vi "ttm_tensilecyclic_poller.vi"() -> ()   [LabVIEW 2011]
panel:
  out "error out":errorcluster
  out "Cycles":i32
  out "Afterramp":i32
  out "Preramp":i32
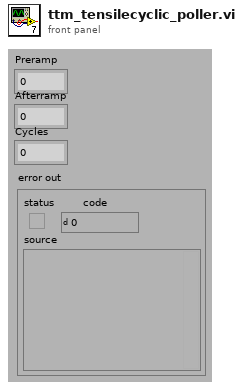
[diagram p1: front panel]
types:
  T1 = cluster{"Name":string, "Type":i32, "SI Full Scale":dbl, "Full Scale":dbl, "Units String":string, "Display Format":string, "Gauge Length":dbl}[][]
  T2 = cluster{"Device ID":i32, "Device Name":string, "Device Type":i32}[]
  T3 = cluster{"Double":dbl, "Set Point Time":dbl, "Double":dbl, "Double":dbl}
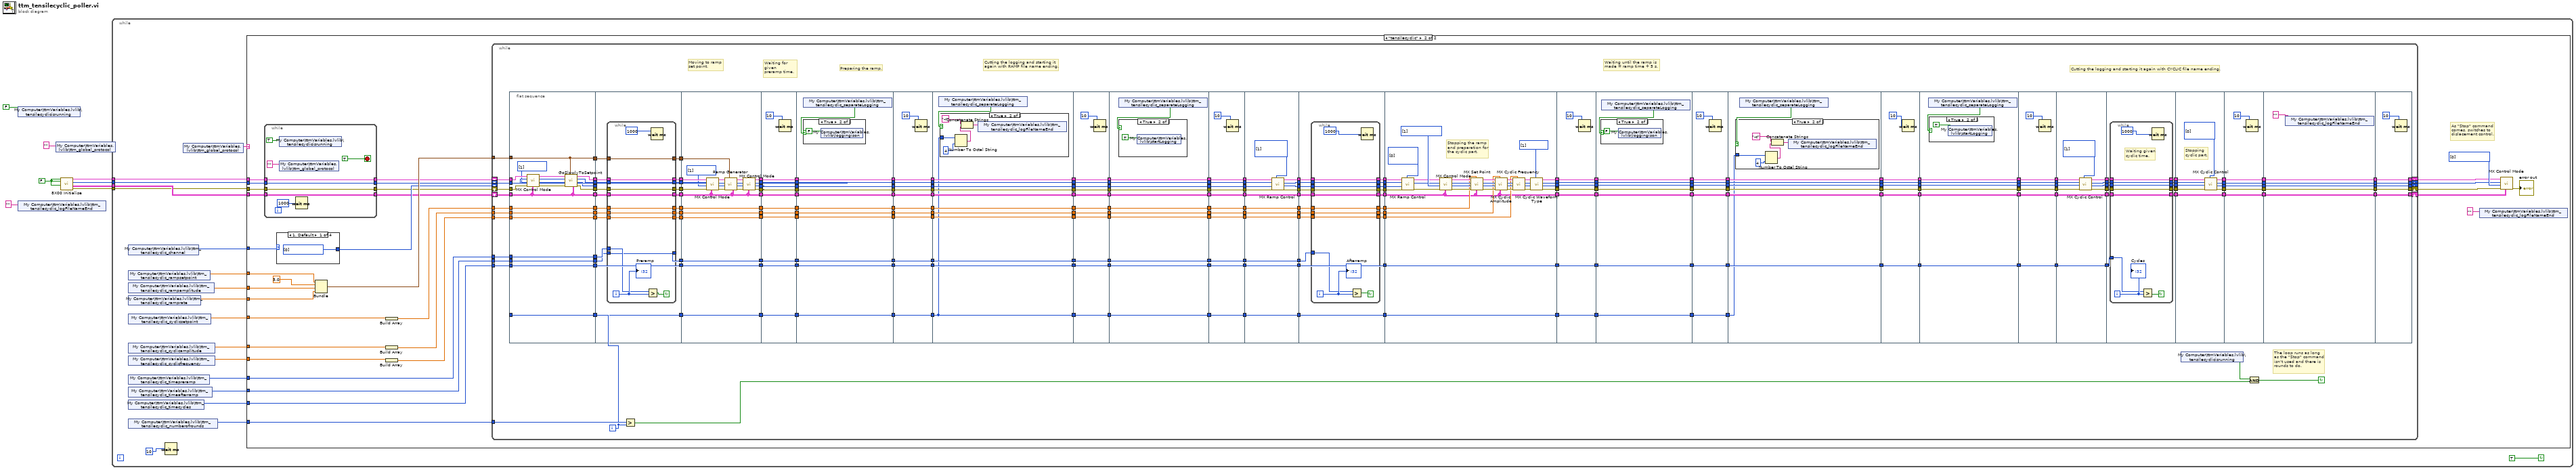
[diagram p0: block diagram]
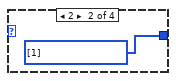
[diagram p9: hidden frame]
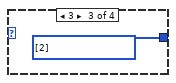
[diagram p10: hidden frame]
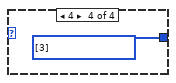
[diagram p11: hidden frame]
diagram:
  w4 = FALSE ("Reset?")
  n1 = shared-variable "My Computer\\ttmVariables.lvlib\\tensilecyclicisrunning"(FALSE ("tensilecyclicisrunning")) -> ()  [unwired: 1 in, 1 out]
  n2 = shared-variable "My Computer\\ttmVariables.lvlib\\ttm_tensilecyclic_logFileNameEnd"("" ("protocol")) -> ()  [unwired: 1 in, 1 out]
  n3 = shared-variable "My Computer\\ttmVariables.lvlib\\ttm_global_protocol"("" ("protocol")) -> ()  [unwired: 1 in, 1 out]
  n4 = call "8X00 Initialise.vi"("Reset?"=w4, "Create DVM? (T)"=w4, "Create Console? (T)"=w4) -> ("error out"=w5:errorcluster, "Channel Data"=w8:T1, "Axis Selector"=w6:i32[], "Axis Information"=w7:T2)  [unwired: 1 in]
  n5 = while {
    tunnel: w8 -> [w24]
    tunnel: w7 -> [w25]
    tunnel: w6 -> [w13]
    tunnel: w5 -> [w23]
    stop <- TRUE continue-if-true
    n6 = shared-variable "My Computer\\ttmVariables.lvlib\\ttm_tensilecyclic_channel"() -> (w19:i32)  [unwired: 1 in, 1 out]
    n7 = shared-variable "My Computer\\ttmVariables.lvlib\\ttm_tensilecyclic_rampsetpoint"() -> (w12:dbl)  [unwired: 1 in, 1 out]
    n8 = shared-variable "My Computer\\ttmVariables.lvlib\\ttm_tensilecyclic_rampamplitude"() -> (w22:dbl)  [unwired: 1 in, 1 out]
    n9 = shared-variable "My Computer\\ttmVariables.lvlib\\ttm_tensilecyclic_ramprate"() -> (w21:dbl)  [unwired: 1 in, 1 out]
    n10 = shared-variable "My Computer\\ttmVariables.lvlib\\ttm_tensilecyclic_cyclicsetpoint"() -> (w17:dbl)  [unwired: 1 in, 1 out]
    n11 = shared-variable "My Computer\\ttmVariables.lvlib\\ttm_tensilecyclic_cyclicamplitude"() -> (w16:dbl)  [unwired: 1 in, 1 out]
    n12 = shared-variable "My Computer\\ttmVariables.lvlib\\ttm_tensilecyclic_cyclicfrequency"() -> (w15:dbl)  [unwired: 1 in, 1 out]
    n13 = shared-variable "My Computer\\ttmVariables.lvlib\\ttm_tensilecyclic_timepreramp"() -> (w11:i32)  [unwired: 1 in, 1 out]
    n14 = shared-variable "My Computer\\ttmVariables.lvlib\\ttm_tensilecyclic_timeafterramp"() -> (w9:i32)  [unwired: 1 in, 1 out]
    n15 = shared-variable "My Computer\\ttmVariables.lvlib\\ttm_tensilecyclic_timecycles"() -> (w10:i32)  [unwired: 1 in, 1 out]
    n16 = shared-variable "My Computer\\ttmVariables.lvlib\\ttm_tensilecyclic_numberofrounds"() -> (w14:i32)  [unwired: 1 in, 1 out]
    n17 = Wait (ms)(milliseconds to wait=u32 10) -> ()  [unwired: 1 out]
    n18 = shared-variable "My Computer\\ttmVariables.lvlib\\ttm_global_protocol"() -> (w18:string)  [unwired: 1 in, 1 out]
    n19 = case shown="\"tensilecyclic\"" w18 {
      tunnel: w13 -> [_ w46]
      tunnel: w25 -> [_ w47]
      tunnel: w24 -> [_ w44]
      tunnel: w23 -> [_ w45]
      tunnel: w22 -> [_ w57]
      tunnel: w21 -> [_ w56]
      tunnel: w19 -> [_ w55]
      tunnel: w17 -> [_ w54]
      tunnel: w16 -> [_ w52]
      tunnel: w15 -> [_ w49]
      tunnel: w14 -> [_ w43]
      tunnel: w12 -> [_ w32]
      tunnel: w11 -> [_ w31]
      tunnel: w10 -> [_ w30]
      tunnel: w9 -> [_ w29]
      frame "", Default {
      }
      frame "tensilecyclic" {
        w37 = u16[] [0] items=["Channel 1", "Channel 2", "Channel 3", "Channel 4"] ("Control Modes")
        # "As \"Stop\" command\ncomes, switches to\ndislacement control."
        n20 = while {
          tunnel: [w62] -> w42
          tunnel: w47 -> [w62]
          tunnel: [w61] -> w41
          tunnel: w46 -> [w61]
          tunnel: [w60] -> w39
          tunnel: w45 -> [w60]
          tunnel: [w59] -> w38
          tunnel: w44 -> [w59]
          stop <- TRUE stop-if-true
          n21 = shared-variable "My Computer\\ttmVariables.lvlib\\tensilecyclicisrunning"(TRUE ("tensilecyclicisrunning")) -> ()  [unwired: 1 in, 1 out]
          n22 = shared-variable "My Computer\\ttmVariables.lvlib\\ttm_global_protocol"("" ("protocol")) -> ()  [unwired: 1 in, 1 out]
          n23 = Wait (ms)(milliseconds to wait=u32 1000) -> ()  [unwired: 1 out]
        }
        n24 = case shown="1, Default" w55 {
          tunnel: [w671 w672 w673 w674] -> w40
          frame 1, Default {
            w671 = u16[] [0] items=["Channel 1", "Channel 2", "Channel 3", "Channel 4"] ("Choose channel to apply\nthe setpoint")
          }
          frame 2 {
            w672 = u16[] [1] items=["Channel 1", "Channel 2", "Channel 3", "Channel 4"] ("Choose channel to apply\nthe setpoint")
          }
          frame 3 {
            w673 = u16[] [2] items=["Channel 1", "Channel 2", "Channel 3", "Channel 4"] ("Choose channel to apply\nthe setpoint")
          }
          frame 4 {
            w674 = u16[] [3] items=["Channel 1", "Channel 2", "Channel 3", "Channel 4"] ("Choose channel to apply\nthe setpoint")
          }
        }
        n25 = Bundle("Double"=w32, "Set Point Time"=3.0, "Double"=w57, "Double"=w56) -> (w58:T3)  [unwired: 1 in]
        n26 = Build Array(w54) -> (w53:dbl[])
        n27 = Build Array(w52) -> (w51:dbl[])
        n28 = Build Array(w49) -> (w48:dbl[])
        n29 = while {
          tunnel: w58 -> [w84]
          tunnel: w53 -> [w79]
          tunnel: w51 -> [w78]
          tunnel: w48 -> [w77]
          tunnel: w43 -> [w298]
          shift-right: [w72] -> w36
          shift-left: w42 -> [w83]
          shift-right: [w71] -> w35
          shift-left: w41 -> [w82]
          shift-right: [w70] -> _
          shift-left: w40 -> [_]
          shift-right: [w69] -> w34
          shift-left: w39 -> [w81]
          shift-right: [w68] -> w33
          shift-left: w38 -> [w80]
          tunnel: w31 -> [w76]
          tunnel: w29 -> [w74]
          tunnel: w30 -> [w73]
          i -> [w75]
          stop <- w67 continue-if-true
          # "Waiting until the ramp is made = ramp time + 5 s."
          # "Moving to ramp\nset point."
          # "Waiting for given\npreramp time."
          # "Preparing the ramp."
          # "Cutting the logging and starting it again with RAMP file name ending."
          # "Cutting the logging and starting it again with CYCLIC file name ending."
          # "The loop runs as long\nas the \"Stop\" command\nisn't used and there is \nrounds to do."
          n30 = flat-sequence {
            tunnel: w84 -> [w303]
            tunnel: w82 -> [w316]
            tunnel: w83 -> [w317]
            tunnel: w79 -> [w319]
            tunnel: w78 -> [w318]
            tunnel: [w319] -> w295
            tunnel: [w318] -> w294
            tunnel: [w310] -> w293
            tunnel: [w309] -> w292
            tunnel: [w308] -> w291
            tunnel: [w307] -> w290
            tunnel: [w304] -> w289
            tunnel: [w303] -> w288
            tunnel: w77 -> [w306]
            tunnel: [w306] -> w287
            tunnel: w81 -> [w305]
            tunnel: w80 -> [w304]
            tunnel: w76 -> [w302]
            tunnel: [w302] -> w286
            tunnel: w74 -> [w301]
            tunnel: [w301] -> w285
            tunnel: w73 -> [w300]
            tunnel: [w300] -> w284
            tunnel: [w299] -> w283
            tunnel: w75 -> [w299]
            tunnel: w295 -> [w330]
            tunnel: [w329] -> w282
            tunnel: w294 -> [w327]
            tunnel: [w328] -> w281
            tunnel: w293 -> [w337]
            tunnel: [w338] -> w280
            tunnel: w292 -> [w336]
            tunnel: [w335] -> w279
            tunnel: w291 -> [_]
            tunnel: w290 -> [w333]
            tunnel: [w334] -> w278
            tunnel: w289 -> [w331]
            tunnel: [w332] -> w277
            tunnel: [w339] -> w276
            tunnel: w288 -> [w340]
            tunnel: [w326] -> w275
            tunnel: w287 -> [w325]
            tunnel: w286 -> [w324]
            tunnel: [w323] -> w274
            tunnel: w285 -> [w322]
            tunnel: w284 -> [w321]
            tunnel: [w321] -> w273
            tunnel: [w320] -> w272
            tunnel: w283 -> [w320]
            tunnel: w282 -> [w377]
            tunnel: [w377] -> w271
            tunnel: w281 -> [w376]
            tunnel: [w376] -> w270
            tunnel: w280 -> [w367]
            tunnel: [w358] -> w269
            tunnel: w279 -> [w366]
            tunnel: [w357] -> w268
            tunnel: [w355] -> w267
            tunnel: w278 -> [w364]
            tunnel: [w356] -> w266
            tunnel: w277 -> [w362]
            tunnel: [w362] -> w265
            tunnel: w276 -> [w363]
            tunnel: w275 -> [w361]
            tunnel: [w361] -> w264
            tunnel: [w360] -> w263
            tunnel: w274 -> [w360]
            tunnel: [w359] -> w262
            tunnel: w273 -> [w359]
            tunnel: [w354] -> w261
            tunnel: w272 -> [w354]
            tunnel: w271 -> [w389]
            tunnel: [w389] -> w260
            tunnel: w270 -> [w388]
            tunnel: [w388] -> w259
            tunnel: w269 -> [w387]
            tunnel: [w387] -> w258
            tunnel: w268 -> [w386]
            tunnel: [w386] -> w257
            tunnel: w267 -> [w385]
            tunnel: [w385] -> w256
            tunnel: w266 -> [w384]
            tunnel: [w384] -> w255
            tunnel: w265 -> [w383]
            tunnel: [w383] -> w254
            tunnel: w264 -> [w382]
            tunnel: [w382] -> w253
            tunnel: w263 -> [w381]
            tunnel: [w381] -> w252
            tunnel: w262 -> [w380]
            tunnel: [w380] -> w251
            tunnel: w261 -> [w379]
            tunnel: [w379] -> w250
            tunnel: w260 -> [w401]
            tunnel: [w401] -> w249
            tunnel: w259 -> [w400]
            tunnel: [w400] -> w248
            tunnel: w258 -> [w399]
            tunnel: [w399] -> w247
            tunnel: w257 -> [w398]
            tunnel: [w398] -> w246
            tunnel: w256 -> [w397]
            tunnel: [w397] -> w245
            tunnel: w255 -> [w396]
            tunnel: [w396] -> w244
            tunnel: w254 -> [w395]
            tunnel: [w395] -> w243
            tunnel: w253 -> [w394]
            tunnel: [w394] -> w242
            tunnel: w252 -> [w393]
            tunnel: [w393] -> w241
            tunnel: w251 -> [w392]
            tunnel: [w392] -> w240
            tunnel: [w391] -> w239
            tunnel: w250 -> [w391]
            tunnel: w249 -> [w414]
            tunnel: [w414] -> w238
            tunnel: w248 -> [w413]
            tunnel: [w413] -> w237
            tunnel: w247 -> [w412]
            tunnel: [w412] -> w236
            tunnel: w246 -> [w411]
            tunnel: [w411] -> w235
            tunnel: w245 -> [w410]
            tunnel: [w410] -> w234
            tunnel: w244 -> [w409]
            tunnel: [w409] -> w233
            tunnel: w243 -> [w408]
            tunnel: [w408] -> w232
            tunnel: w242 -> [w407]
            tunnel: [w407] -> w231
            tunnel: w241 -> [w406]
            tunnel: [w406] -> w230
            tunnel: w240 -> [w405]
            tunnel: [w405] -> w229
            tunnel: [w404] -> w228
            tunnel: w239 -> [w404]
            tunnel: w238 -> [w426]
            tunnel: [w426] -> w227
            tunnel: w237 -> [w425]
            tunnel: [w425] -> w226
            tunnel: w236 -> [w424]
            tunnel: [w424] -> w225
            tunnel: w235 -> [w423]
            tunnel: [w423] -> w224
            tunnel: w234 -> [w422]
            tunnel: [w422] -> w223
            tunnel: w233 -> [w421]
            tunnel: [w421] -> w222
            tunnel: w232 -> [w420]
            tunnel: [w420] -> w221
            tunnel: w231 -> [w419]
            tunnel: [w419] -> w220
            tunnel: w230 -> [w418]
            tunnel: [w418] -> w219
            tunnel: w229 -> [w417]
            tunnel: [w417] -> w218
            tunnel: w228 -> [w415]
            tunnel: [w415] -> w217
            tunnel: w227 -> [w443]
            tunnel: [w443] -> w216
            tunnel: w226 -> [w442]
            tunnel: [w442] -> w215
            tunnel: w225 -> [w441]
            tunnel: [w441] -> w214
            tunnel: w224 -> [w440]
            tunnel: [w440] -> w213
            tunnel: w223 -> [w439]
            tunnel: [w439] -> w212
            tunnel: w222 -> [w438]
            tunnel: [w438] -> w211
            tunnel: w221 -> [w437]
            tunnel: [w437] -> w210
            tunnel: w220 -> [w436]
            tunnel: [w436] -> w209
            tunnel: w219 -> [w435]
            tunnel: [w435] -> w208
            tunnel: w218 -> [w434]
            tunnel: [w434] -> w207
            tunnel: [w433] -> w206
            tunnel: w217 -> [w433]
            tunnel: w216 -> [w455]
            tunnel: [w455] -> w205
            tunnel: w215 -> [w454]
            tunnel: [w454] -> w204
            tunnel: w214 -> [w453]
            tunnel: [w453] -> w203
            tunnel: w213 -> [w452]
            tunnel: [w452] -> w202
            tunnel: w212 -> [w451]
            tunnel: [w451] -> w201
            tunnel: w211 -> [w450]
            tunnel: [w450] -> w200
            tunnel: w210 -> [w449]
            tunnel: [w449] -> w199
            tunnel: w209 -> [w448]
            tunnel: [w448] -> w198
            tunnel: w208 -> [w447]
            tunnel: [w447] -> w197
            tunnel: w207 -> [w446]
            tunnel: [w446] -> w196
            tunnel: [w445] -> w195
            tunnel: w206 -> [w445]
            tunnel: w205 -> [w468]
            tunnel: [w468] -> w194
            tunnel: w204 -> [w467]
            tunnel: [w467] -> w193
            tunnel: w203 -> [w466]
            tunnel: [w466] -> w192
            tunnel: w202 -> [w465]
            tunnel: [w465] -> w191
            tunnel: w201 -> [w464]
            tunnel: [w464] -> w190
            tunnel: w200 -> [w463]
            tunnel: [w463] -> w189
            tunnel: w199 -> [w462]
            tunnel: [w462] -> w188
            tunnel: w198 -> [w461]
            tunnel: [w461] -> w187
            tunnel: w197 -> [w460]
            tunnel: [w460] -> w186
            tunnel: w196 -> [w459]
            tunnel: [w459] -> w185
            tunnel: [w458] -> w184
            tunnel: w195 -> [w458]
            tunnel: w194 -> [w484]
            tunnel: [w484] -> w183
            tunnel: w193 -> [w483]
            tunnel: [w483] -> w182
            tunnel: w192 -> [w471]
            tunnel: [w478] -> w181
            tunnel: w191 -> [w472]
            tunnel: [w477] -> w180
            tunnel: w190 -> [w473]
            tunnel: [w476] -> w179
            tunnel: w189 -> [w474]
            tunnel: [w475] -> w178
            tunnel: w188 -> [w470]
            tunnel: [w470] -> w177
            tunnel: w187 -> [w482]
            tunnel: [w482] -> w176
            tunnel: w186 -> [w481]
            tunnel: [w481] -> w175
            tunnel: w185 -> [w480]
            tunnel: [w480] -> w174
            tunnel: [w469] -> w173
            tunnel: w184 -> [w469]
            tunnel: [w493] -> w172
            tunnel: w183 -> [w492]
            tunnel: [w491] -> w171
            tunnel: w182 -> [w490]
            tunnel: [w503] -> w170
            tunnel: w181 -> [w502]
            tunnel: [w501] -> w169
            tunnel: w180 -> [w500]
            tunnel: [w499] -> w168
            tunnel: w179 -> [w498]
            tunnel: [w497] -> w167
            tunnel: w178 -> [w496]
            tunnel: [w495] -> w166
            tunnel: w177 -> [w494]
            tunnel: [w488] -> w165
            tunnel: w176 -> [w489]
            tunnel: w175 -> [w487]
            tunnel: w174 -> [w486]
            tunnel: [w486] -> w164
            tunnel: [w485] -> w163
            tunnel: w173 -> [w485]
            tunnel: w172 -> [w546]
            tunnel: w171 -> [w529]
            tunnel: w170 -> [w545]
            tunnel: w169 -> [w544]
            tunnel: w168 -> [w543]
            tunnel: w167 -> [w542]
            tunnel: w166 -> [w523]
            tunnel: [w519] -> w162
            tunnel: [w518] -> w161
            tunnel: [w517] -> w160
            tunnel: [w516] -> w159
            tunnel: w165 -> [w524]
            tunnel: [w523] -> w158
            tunnel: w164 -> [w522]
            tunnel: [w522] -> w157
            tunnel: [w520] -> w156
            tunnel: w163 -> [w520]
            tunnel: w162 -> [w559]
            tunnel: [w559] -> w155
            tunnel: w161 -> [w558]
            tunnel: [w558] -> w154
            tunnel: w160 -> [w557]
            tunnel: [w557] -> w153
            tunnel: w159 -> [w556]
            tunnel: [w556] -> w152
            tunnel: w158 -> [w555]
            tunnel: [w555] -> w151
            tunnel: w157 -> [w554]
            tunnel: [w554] -> w150
            tunnel: w156 -> [w553]
            tunnel: [w553] -> w149
            tunnel: w155 -> [w567]
            tunnel: [w567] -> w148
            tunnel: w154 -> [w566]
            tunnel: [w566] -> w147
            tunnel: w153 -> [w565]
            tunnel: [w565] -> w146
            tunnel: w152 -> [w564]
            tunnel: [w564] -> w145
            tunnel: w151 -> [w563]
            tunnel: [w563] -> w144
            tunnel: w150 -> [w562]
            tunnel: [w562] -> w143
            tunnel: w149 -> [w561]
            tunnel: [w561] -> w142
            tunnel: w148 -> [w576]
            tunnel: [w576] -> w141
            tunnel: w147 -> [w575]
            tunnel: [w575] -> w140
            tunnel: w146 -> [w574]
            tunnel: [w574] -> w139
            tunnel: w145 -> [w573]
            tunnel: [w573] -> w138
            tunnel: w144 -> [w572]
            tunnel: [w572] -> w137
            tunnel: w143 -> [w571]
            tunnel: [w571] -> w136
            tunnel: w142 -> [w570]
            tunnel: [w570] -> w135
            tunnel: w141 -> [w584]
            tunnel: [w584] -> w134
            tunnel: w140 -> [w583]
            tunnel: [w583] -> w133
            tunnel: w139 -> [w582]
            tunnel: [w582] -> w132
            tunnel: w138 -> [w581]
            tunnel: [w581] -> w131
            tunnel: w137 -> [w580]
            tunnel: [w580] -> w130
            tunnel: w136 -> [w579]
            tunnel: [w579] -> w129
            tunnel: w135 -> [w577]
            tunnel: w134 -> [w596]
            tunnel: [w596] -> w128
            tunnel: w133 -> [w595]
            tunnel: [w595] -> w127
            tunnel: w132 -> [w594]
            tunnel: [w594] -> w126
            tunnel: w131 -> [w593]
            tunnel: [w593] -> w125
            tunnel: w130 -> [w592]
            tunnel: [w592] -> w124
            tunnel: w129 -> [w591]
            tunnel: [w591] -> w123
            tunnel: w128 -> [w603]
            tunnel: [w603] -> w122
            tunnel: w127 -> [w602]
            tunnel: [w602] -> w121
            tunnel: w126 -> [w601]
            tunnel: [w601] -> w120
            tunnel: w125 -> [w600]
            tunnel: [w600] -> w119
            tunnel: w124 -> [w599]
            tunnel: [w599] -> w118
            tunnel: w123 -> [w598]
            tunnel: [w598] -> w117
            tunnel: w122 -> [w611]
            tunnel: [w611] -> w116
            tunnel: w121 -> [w610]
            tunnel: [w610] -> w115
            tunnel: w120 -> [w609]
            tunnel: [w609] -> w114
            tunnel: w119 -> [w608]
            tunnel: [w608] -> w113
            tunnel: w118 -> [w607]
            tunnel: [w607] -> w112
            tunnel: w117 -> [w606]
            tunnel: [w606] -> w111
            tunnel: w116 -> [w617]
            tunnel: [w619] -> w110
            tunnel: w115 -> [w616]
            tunnel: [w618] -> w109
            tunnel: w114 -> [w615]
            tunnel: w113 -> [w614]
            tunnel: [w612] -> w108
            tunnel: w112 -> [w622]
            tunnel: [w622] -> w107
            tunnel: w111 -> [w621]
            tunnel: [w621] -> w106
            tunnel: [w613] -> w105
            tunnel: w110 -> [w632]
            tunnel: [w633] -> w104
            tunnel: [w631] -> w103
            tunnel: w109 -> [w630]
            tunnel: [w629] -> w102
            tunnel: [w627] -> w101
            tunnel: w108 -> [w626]
            tunnel: [w625] -> w100
            tunnel: w107 -> [w624]
            tunnel: w106 -> [w623]
            tunnel: w105 -> [w628]
            tunnel: w104 -> [w652]
            tunnel: w103 -> [w651]
            tunnel: w102 -> [w650]
            tunnel: w101 -> [w649]
            tunnel: w100 -> [w643]
            tunnel: [w647] -> w99
            tunnel: [w646] -> w98
            tunnel: [w645] -> w97
            tunnel: [w644] -> w96
            tunnel: [w643] -> w95
            tunnel: w99 -> [w658]
            tunnel: w98 -> [w657]
            tunnel: w97 -> [w656]
            tunnel: w96 -> [w655]
            tunnel: w95 -> [w654]
            tunnel: [w658] -> w94
            tunnel: [w657] -> w93
            tunnel: [w656] -> w92
            tunnel: [w655] -> w91
            tunnel: [w654] -> w90
            tunnel: w94 -> [w664]
            tunnel: w93 -> [w663]
            tunnel: w92 -> [w662]
            tunnel: w91 -> [w661]
            tunnel: w90 -> [w660]
            tunnel: [w664] -> w89
            tunnel: [w663] -> w88
            tunnel: [w662] -> w87
            tunnel: [w661] -> w86
            tunnel: [w660] -> w85
            tunnel: [w666] -> w68
            tunnel: [w667] -> w69
            tunnel: [w668] -> w70
            tunnel: [w669] -> w71
            tunnel: [w670] -> w72
            tunnel: w89 -> [w670]
            tunnel: w88 -> [w669]
            tunnel: w87 -> [w668]
            tunnel: w86 -> [w667]
            tunnel: w85 -> [w666]
            frame #0 {
              w311 = u16[] [1] items=["Channel 1", "Channel 2", "Channel 3", "Channel 4"] ("Control Modes")
              n31 = call "MX Control Mode.vi"("Channel Data"=w304, "error in (no error)"=w305, "Control Modes"=w311, "Axis Selector"=w316, "Axis Information"=w317) -> ("error out"=w315:errorcluster, "Control Modes out"=w314:u16[], "Axis Selector out"=w313:i32[], "Axis Information out"=w312:T2)  [unwired: 1 in]
              n32 = call "GoSlowlyToSetpoint.vi"("Channel Data"=w304, "Input cluster"=w303, "error in (no error)"=w315, "Channels"=w314, "Axis Selector"=w313, "Axis Information"=w312) -> ("Error Out"=w307:errorcluster, "Channels Out"=w308:u16[], "Axis Selector Out"=w309:i32[], "Axis Information Out"=w310:T2)  [unwired: 2 in]
            }
            frame #1 {
              n33 = while {
                tunnel: w340 -> [w352]
                tunnel: [w352] -> w339
                tunnel: [w351] -> w338
                tunnel: w337 -> [w351]
                tunnel: w336 -> [w350]
                tunnel: [w350] -> w335
                tunnel: [w349] -> w334
                tunnel: w333 -> [w349]
                tunnel: [w348] -> w332
                tunnel: w331 -> [w348]
                tunnel: [w347] -> w329
                tunnel: w330 -> [w347]
                tunnel: [w346] -> w328
                tunnel: w327 -> [w346]
                tunnel: [w345] -> w326
                tunnel: w325 -> [w345]
                tunnel: w324 -> [w342]
                tunnel: [w341] -> w323
                tunnel: w322 -> [w341]
                i -> [w343]
                stop <- w344 continue-if-true
                n34 = Greater?(x=w342, y=w343) -> (0:w344:bool)
                n35 = Wait (ms)(milliseconds to wait=u32 1000) -> ()  [unwired: 1 out]
                "Preramp" <- w343
              }
            }
            frame #2 {
              w365 = u16[] [1] items=["Channel 1", "Channel 2", "Channel 3", "Channel 4"] ("Control Modes")
              n36 = call "MX Control Mode.vi"("Channel Data"=w362, "error in (no error)"=w364, "Control Modes"=w365, "Axis Selector"=w366, "Axis Information"=w367) -> ("error out"=w368:errorcluster, "Control Modes out"=w369:u16[], "Axis Selector out"=w370:i32[], "Axis Information out"=w371:T2)  [unwired: 1 in]
              n37 = call "Ramp Generator.vi"("Channel Data"=w362, "Input cluster"=w363, "error in (no error)"=w368, "Channels"=w369, "Axis Selector"=w370, "Axis Information"=w371) -> ("Error Out"=w372:errorcluster, "Channels Out"=w373:u16[], "Axis Selector Out"=w374:i32[], "Axis Information Out"=w375:T2)  [unwired: 2 in]
              n38 = call "MX Control Mode.vi"("Channel Data"=w362, "error in (no error)"=w372, "Control Modes"=w373, "Axis Selector"=w374, "Axis Information"=w375) -> ("error out"=w356:errorcluster, "Control Modes out"=w355:u16[], "Axis Selector out"=w357:i32[], "Axis Information out"=w358:T2)  [unwired: 1 in]
            }
            frame #3 {
              n39 = Wait (ms)(milliseconds to wait=u32 10) -> ()  [unwired: 1 out]
            }
            frame #4 {
              n40 = shared-variable "My Computer\\ttmVariables.lvlib\\ttm_tensilecyclic_separateLogging"() -> (w390:bool)  [unwired: 1 in, 1 out]
              n41 = case shown="True" w390 {
                frame False {
                }
                frame True {
                  n42 = shared-variable "My Computer\\ttmVariables.lvlib\\loggingison"(FALSE ("tensilecyclicisrunning")) -> ()  [unwired: 1 in, 1 out]
                }
              }
            }
            frame #5 {
              n43 = Wait (ms)(milliseconds to wait=u32 10) -> ()  [unwired: 1 out]
            }
            frame #6 {
              n44 = shared-variable "My Computer\\ttmVariables.lvlib\\ttm_tensilecyclic_separateLogging"() -> (w416:bool)  [unwired: 1 in, 1 out]
              n45 = case shown="True" w416 {
                tunnel: w415 -> [_ w427]
                frame False {
                }
                frame True {
                  n46 = Number To Octal String(1:4, 2:w427) -> (0:w430:string)
                  n47 = Concatenate Strings("-r", w430) -> (w428:string)
                  n48 = shared-variable "My Computer\\ttmVariables.lvlib\\ttm_tensilecyclic_logFileNameEnd"(w428) -> ()  [unwired: 1 in, 1 out]
                }
              }
            }
            frame #7 {
              n49 = Wait (ms)(milliseconds to wait=u32 10) -> ()  [unwired: 1 out]
            }
            frame #8 {
              n50 = shared-variable "My Computer\\ttmVariables.lvlib\\ttm_tensilecyclic_separateLogging"() -> (w444:bool)  [unwired: 1 in, 1 out]
              n51 = case shown="True" w444 {
                frame False {
                }
                frame True {
                  n52 = shared-variable "My Computer\\ttmVariables.lvlib\\startLogging"(TRUE ("tensilecyclicisrunning")) -> ()  [unwired: 1 in, 1 out]
                }
              }
            }
            frame #9 {
              n53 = Wait (ms)(milliseconds to wait=u32 10) -> ()  [unwired: 1 out]
            }
            frame #10 {
              w479 = u16[] [1] items=["Stop", "Start or continue", "Hold", "Continue", "Return ramp to set level at fixed rate", "Reserved", "Reserved", "Start Random without demand hold", "Start Random with demand hold", "Prepare Random Start without demand hold", "Prepare Random Start with demand hold", "Unslave", "Reserved", "Reserved", "Start Sample Data Playback or Resume", "Prepare for Start of Sample Data", "Reserved", "Reserved", "Resume Playback", "Start an electromechanical frame return"] ("Ramp Control")
              n54 = call "MX Ramp Control.vi"("Ramp Control"=w479, "error in (no error)"=w474, "Channels In"=w473, "Axis Selector In"=w472, "Axis Information In"=w471) -> ("error out"=w475:errorcluster, "Channels Out"=w476:u16[], "Axis Selector Out"=w477:i32[], "Axis Information Out"=w478:T2)  [unwired: 2 in]
            }
            frame #11 {
              n55 = while {
                tunnel: [w514] -> w503
                tunnel: w502 -> [w514]
                tunnel: [w513] -> w501
                tunnel: w500 -> [w513]
                tunnel: [w512] -> w499
                tunnel: w498 -> [w512]
                tunnel: [w511] -> w497
                tunnel: w496 -> [w511]
                tunnel: [w510] -> w495
                tunnel: w494 -> [w510]
                tunnel: [w509] -> w493
                tunnel: w492 -> [w509]
                tunnel: [w508] -> w491
                tunnel: w490 -> [w508]
                tunnel: w489 -> [w507]
                tunnel: [w507] -> w488
                tunnel: w487 -> [w504]
                i -> [w505]
                stop <- w506 continue-if-true
                n56 = Greater?(x=w504, y=w505) -> (0:w506:bool)
                n57 = Wait (ms)(milliseconds to wait=u32 1000) -> ()  [unwired: 1 out]
                "Afterramp" <- w505
              }
            }
            frame #12 {
              w528 = u16[] [1] items=["Channel 1", "Channel 2", "Channel 3", "Channel 4"] ("Control Modes")
              w521 = u16[] [1] items=["Sine", "Triangle", "Square", "Haversine", "Havertriangle", "Haversquare", "External - Sensor", "External - Auxillary", "Sawtooth"] ("Waveform Types")
              w547 = u16[] [0] items=["Stop", "Start or continue", "Hold", "Continue", "Return ramp to set level at fixed rate", "Reserved", "Reserved", "Start Random without demand hold", "Start Random with demand hold", "Prepare Random Start without demand hold", "Prepare Random Start with demand hold", "Unslave", "Reserved", "Reserved", "Start Sample Data Playback or Resume", "Prepare for Start of Sample Data", "Reserved", "Reserved", "Resume Playback", "Start an electromechanical frame return"] ("Ramp Control")
              # "Stopping the ramp \nand preparation for\nthe cyclic part."
              n58 = call "MX Ramp Control.vi"("Ramp Control"=w547, "error in (no error)"=w542, "Channels In"=w543, "Axis Selector In"=w544, "Axis Information In"=w545) -> ("error out"=w525:errorcluster, "Axis Selector Out"=w526:i32[], "Axis Information Out"=w527:T2)  [unwired: 2 in, 1 out]
              n59 = call "MX Control Mode.vi"("Channel Data"=w523, "error in (no error)"=w525, "Control Modes"=w528, "Axis Selector"=w526, "Axis Information"=w527) -> ("error out"=w551:errorcluster, "Control Modes out"=w550:u16[], "Axis Selector out"=w549:i32[], "Axis Information out"=w548:T2)  [unwired: 1 in]
              n60 = call "MX Set Point.vi"("Channel Data"=w523, "Set Point"=w546, "error in (no error)"=w551, "Channels"=w550, "Axis Selector"=w549, "Axis Information"=w548) -> ("error out"=w530:errorcluster, "Channels out"=w531:u16[], "Axis Selector out"=w532:i32[], "Axis Information out"=w533:T2)
              n61 = call "MX Cyclic Amplitude.vi"("Channel Data"=w523, "Cyclic Amplitude"=w529, "error in (no error)"=w530, "Channels"=w531, "Axis Selector"=w532, "Axis Information"=w533) -> ("error out"=w541:errorcluster, "Channels out"=w540:u16[], "Axis Selector out"=w539:i32[], "Axis Information out"=w538:T2)  [unwired: 1 in]
              n62 = call "MX Cyclic Frequency.vi"("Cyclic Frequency"=w524, "error in (no error)"=w541, "Channels"=w540, "Axis Selector"=w539, "Axis Information"=w538) -> ("error out"=w534:errorcluster, "Channels out"=w535:u16[], "Axis Selector out"=w536:i32[], "Axis Information out"=w537:T2)  [unwired: 2 in]
              n63 = call "MX Cyclic Waveform Type.vi"("Waveform Types"=w521, "error in (no error)"=w534, "Channels"=w535, "Axis Selector"=w536, "Axis Information"=w537) -> ("error out"=w516:errorcluster, "Channels out"=w517:u16[], "Axis Selector out"=w518:i32[], "Axis Information out"=w519:T2)  [unwired: 2 in]
            }
            frame #13 {
              n64 = Wait (ms)(milliseconds to wait=u32 10) -> ()  [unwired: 1 out]
            }
            frame #14 {
              n65 = shared-variable "My Computer\\ttmVariables.lvlib\\ttm_tensilecyclic_separateLogging"() -> (w560:bool)  [unwired: 1 in, 1 out]
              n66 = case shown="True" w560 {
                frame False {
                }
                frame True {
                  n67 = shared-variable "My Computer\\ttmVariables.lvlib\\loggingison"(FALSE ("tensilecyclicisrunning")) -> ()  [unwired: 1 in, 1 out]
                }
              }
            }
            frame #15 {
              n68 = Wait (ms)(milliseconds to wait=u32 10) -> ()  [unwired: 1 out]
            }
            frame #16 {
              n69 = shared-variable "My Computer\\ttmVariables.lvlib\\ttm_tensilecyclic_separateLogging"() -> (w578:bool)  [unwired: 1 in, 1 out]
              n70 = case shown="True" w578 {
                tunnel: w577 -> [_ w585]
                frame False {
                }
                frame True {
                  n71 = Number To Octal String(1:4, 2:w585) -> (0:w588:string)
                  n72 = Concatenate Strings("-c", w588) -> (w586:string)
                  n73 = shared-variable "My Computer\\ttmVariables.lvlib\\ttm_tensilecyclic_logFileNameEnd"(w586) -> ()  [unwired: 1 in, 1 out]
                }
              }
            }
            frame #17 {
              n74 = Wait (ms)(milliseconds to wait=u32 10) -> ()  [unwired: 1 out]
            }
            frame #18 {
              n75 = shared-variable "My Computer\\ttmVariables.lvlib\\ttm_tensilecyclic_separateLogging"() -> (w597:bool)  [unwired: 1 in, 1 out]
              n76 = case shown="True" w597 {
                frame False {
                }
                frame True {
                  n77 = shared-variable "My Computer\\ttmVariables.lvlib\\startLogging"(TRUE ("tensilecyclicisrunning")) -> ()  [unwired: 1 in, 1 out]
                }
              }
            }
            frame #19 {
              n78 = Wait (ms)(milliseconds to wait=u32 10) -> ()  [unwired: 1 out]
            }
            frame #20 {
              w620 = u16[] [1] items=["Stop", "Start or continue", "Hold", "Continue", "Finish current cycle & stop", "Smooth Stop", "Reserved", "Reserved", "Reserved", "Reserved", "Reserved", "Reserved", "Disable", "Enable", "Reserved", "Reserved", "Start/Continue swept waveform", "Dwell at swept frequency"] ("Cyclic Control")
              n79 = call "MX Cyclic Control.vi"("Cyclic Control"=w620, "error in (no error)"=w614, "Channels"=w615, "Axis Selector"=w616, "Axis Information"=w617) -> ("error out"=w612:errorcluster, "Channels out"=w613:u16[], "Axis Selector out"=w618:i32[], "Axis Information out"=w619:T2)  [unwired: 2 in]
            }
            frame #21 {
              n80 = while {
                tunnel: [w641] -> w633
                tunnel: w632 -> [w641]
                tunnel: [w640] -> w631
                tunnel: w630 -> [w640]
                tunnel: [w639] -> w629
                tunnel: w628 -> [w639]
                tunnel: [w638] -> w627
                tunnel: w626 -> [w638]
                tunnel: [w637] -> w625
                tunnel: w624 -> [w637]
                tunnel: w623 -> [w634]
                i -> [w636]
                stop <- w635 continue-if-true
                # "Waiting given\ncyclic time."
                n81 = Greater?(x=w634, y=w636) -> (0:w635:bool)
                n82 = Wait (ms)(milliseconds to wait=u32 1000) -> ()  [unwired: 1 out]
                "Cycles" <- w636
              }
            }
            frame #22 {
              w648 = u16[] [0] items=["Stop", "Start or continue", "Hold", "Continue", "Finish current cycle & stop", "Smooth Stop", "Reserved", "Reserved", "Reserved", "Reserved", "Reserved", "Reserved", "Disable", "Enable", "Reserved", "Reserved", "Start/Continue swept waveform", "Dwell at swept frequency"] ("Cyclic Control")
              # "Stopping\ncyclic part."
              n83 = call "MX Cyclic Control.vi"("Cyclic Control"=w648, "error in (no error)"=w649, "Channels"=w650, "Axis Selector"=w651, "Axis Information"=w652) -> ("error out"=w644:errorcluster, "Channels out"=w645:u16[], "Axis Selector out"=w646:i32[], "Axis Information out"=w647:T2)  [unwired: 2 in]
            }
            frame #23 {
              n84 = Wait (ms)(milliseconds to wait=u32 10) -> ()  [unwired: 1 out]
            }
            frame #24 {
              n85 = shared-variable "My Computer\\ttmVariables.lvlib\\ttm_tensilecyclic_logFileNameEnd"("") -> ()  [unwired: 1 in, 1 out]
            }
            frame #25 {
              n86 = Wait (ms)(milliseconds to wait=u32 10) -> ()  [unwired: 1 out]
            }
          }
          n87 = Greater?(x=w298, y=w75) -> (0:w297:bool)
          n88 = shared-variable "My Computer\\ttmVariables.lvlib\\tensilecyclicisrunning"() -> (w296:bool)  [unwired: 1 in, 1 out]
          n89 = And(x=w296, y=w297) -> (x .and. y?=w67:bool)
        }
        n90 = shared-variable "My Computer\\ttmVariables.lvlib\\ttm_tensilecyclic_logFileNameEnd"("" ("protocol")) -> ()  [unwired: 1 in, 1 out]
        n91 = call "MX Control Mode.vi"("Channel Data"=w33, "error in (no error)"=w34, "Control Modes"=w37, "Axis Selector"=w35, "Axis Information"=w36) -> ("error out"=→"error out":errorcluster)  [unwired: 1 in, 3 out]
      }
    }
  }
